vi "SR830-config.vi"(8 "error in (no error)":errorcluster, 11 "SR830":refnum<vi>) -> (0 "error out":errorcluster)   [LabVIEW 2016]
uses:
  <instrlib>/Stanford Research 830/Stanford Research 830.lvlib
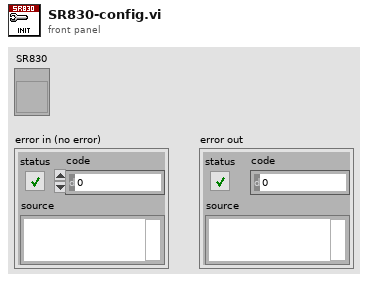
[diagram p1: front panel]
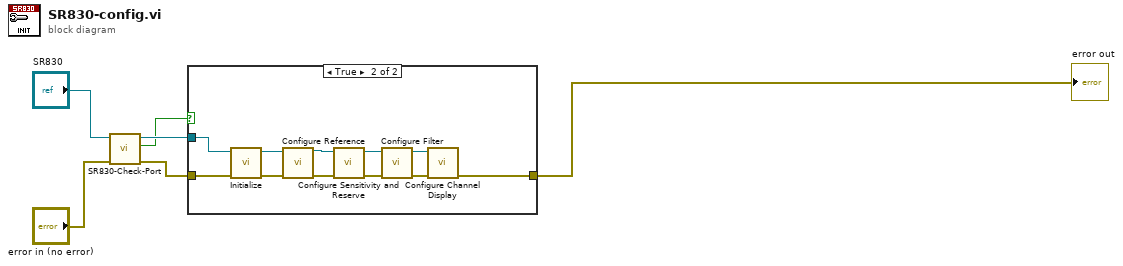
[diagram p0: block diagram]
diagram:
  n1 = call "SR830-Check-Port.vi"("error in (no error)"="error in (no error)", "SR830 in"="SR830") -> ("error out"=w4:errorcluster, "Boolean"=w2:bool, "Sr830 out"=w3:refnum<vi>)  [unwired: 7 in]
  n2 = case shown="True" w2 {
    tunnel: w3 -> [_ w18]
    tunnel: w4 -> [w7 w17]
    tunnel: [w7 w8] -> w5
    frame False {
    }
    frame True {
      n3 = call <instrlib>:"Initialize.vi"("error in (no error)"=w17, "SR830 in"=w18) -> ("error out"=w15:errorcluster, "Sr830 out"=w16:refnum<vi>)  [unwired: 8 in]
      n4 = call <instrlib>:"Configure Reference.vi"("SR830 in"=w16, "error in (no error)"=w15) -> ("Sr830 out"=w13:refnum<vi>, "error out"=w14:errorcluster)  [unwired: 12 in]
      n5 = call <instrlib>:"Configure Sensitivity and Reserve.vi"("error in"=w14, "SR830 in"=w13) -> ("error out"=w11:errorcluster, "Sr830 out"=w12:refnum<vi>)  [unwired: 8 in]
      n6 = call <instrlib>:"Configure Filter.vi"("error in"=w11, "SR830 in"=w12) -> ("error out"=w9:errorcluster, "Sr830 out"=w10:refnum<vi>)  [unwired: 8 in]
      n7 = call <instrlib>:"Configure Channel Display.vi"("error in"=w9, "SR830 in"=w10) -> ("error out"=w8:errorcluster)  [unwired: 8 in, 1 out]
    }
  }
  "error out" <- w5
